vi "Collision Main.vi"() -> (2 "x+y":dbl)   [LabVIEW 2016]
uses:
  <vilib>/Rock Robotics/Network Tables/SD Write Boolean.vi
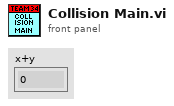
[diagram p1: front panel]
types:
  T1 = cluster{"LinearAcceleration X":dbl, "LinearAcceleration Y":dbl, "LinearAcceleration Z":dbl}
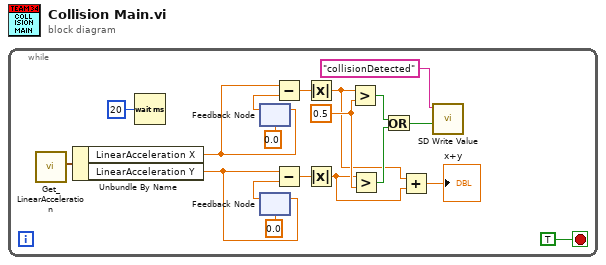
[diagram p0: block diagram]
diagram:
  n1 = while {
    stop <- TRUE stop-if-true
    w10 = 0.5
    n2 = call <vilib>:"Get_LinearAcceleration.vi"() -> ("Linear Acceleration"=w8:T1)  [unwired: 11 in]
    n3 = Unbundle By Name(w8) -> ("LinearAcceleration X"=w16:dbl, "LinearAcceleration Y"=w9:dbl)
    n4 = Wait (ms)(milliseconds to wait=u32 20) -> ()  [unwired: 1 out]
    n5 = feedback #1(0.0) -> (w17:dbl)
    n6 = feedback-in #1(w16) -> ()
    n7 = feedback #2(0.0) -> (w15:dbl)
    n8 = feedback-in #2(w9) -> ()
    n9 = Subtract(x=w16, y=w17) -> (x-y=w18:dbl)
    n10 = Subtract(x=w9, y=w15) -> (x-y=w14:dbl)
    n11 = Absolute Value(x=w18) -> (abs(x)=w4:dbl)
    n12 = Absolute Value(x=w14) -> (abs(x)=w3:dbl)
    n13 = Greater?(x=w4, y=w10) -> (0:w12:bool)
    n14 = Greater?(x=w3, y=w10) -> (0:w11:bool)
    n15 = Or(x=w12, y=w11) -> (x .or. y?=w6:bool)
    n16 = Add(x=w4, y=w3) -> (x+y=→"x+y":dbl)
    n17 = call-poly <vilib>:"SD Write Value.vi"("Boolean"=w6, "Name"="collisionDetected") -> ()  [unwired: 8 in, 2 out]
  }
